vi "PXI_acq.vi"(10 "Sampels/Ch":i32, 11 "Tasks":refnum<k21>[](array[refnum])) -> (3 "Data":dbl[][][](array[numeric]))   [LabVIEW 2013]
uses:
  <vilib>/DAQmx/read.llb/DAQmx Read (Analog 2D DBL NChan NSamp).vi
  <vilib>/DAQmx/miscellaneous.llb/DAQmx Fill In Error Info.vi
  <resource>/objmgr/daqmx.rc
panel:
  out "CurrReadPos 2":dbl=1024.0
  out "AvailSampPerChan 2":u32
  out "TotalSampPerChanAcquired 2":dbl=1024.0
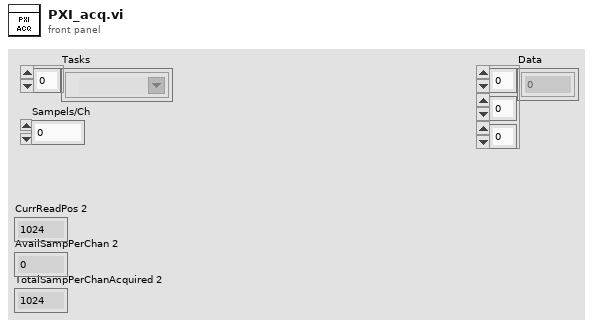
[diagram p1: front panel]
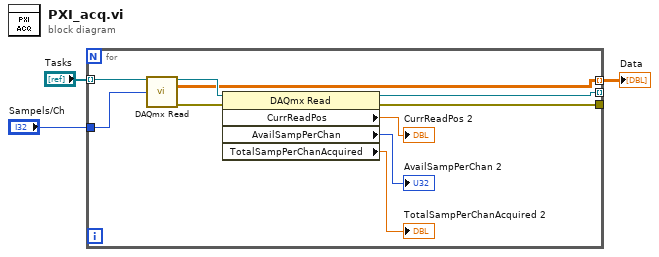
[diagram p0: block diagram]
diagram:
  n1 = for {
    tunnel: [w10] -> _ mode=indexing
    tunnel: "Tasks" -> [w5] mode=indexing
    tunnel: [w7] -> _
    tunnel: "Sampels/Ch" -> [w6]
    tunnel: [w4] -> w1 mode=indexing
    n2 = call-poly <vilib>:"DAQmx Read.vi"("task/channels in"=w5, "number of samples per channel"=w6) -> ("task out"=w11:refnum<k21>, "data"=w4:dbl[][], "error out"=w8:errorcluster)  [unwired: 2 in, 9 out]
    n3 = property class="DAQmx Read"(reference=w11, error in=w8) -> (reference out=w10:refnum<k21>, error out=w7:errorcluster, "CurrReadPos"=→"CurrReadPos 2":dbl, "AvailSampPerChan"=→"AvailSampPerChan 2":u32, "TotalSampPerChanAcquired"=→"TotalSampPerChanAcquired 2":dbl)
  }
  "Data" <- w1
